vi "自动测试计算误差.vi"(8 "反馈值":dbl, 9 "输入值":dbl, 11 "DSP_OR_AD":i32) -> (1 "误差":dbl, 3 "合格？":bool)   [LabVIEW 2010]
uses:
  全局量/全局_配置.vi
panel:
  in  "AD量程":dbl
  in  "误差合格范围":dbl
  in  "DSP量程":dbl
  # "0为DSP，1为AD"
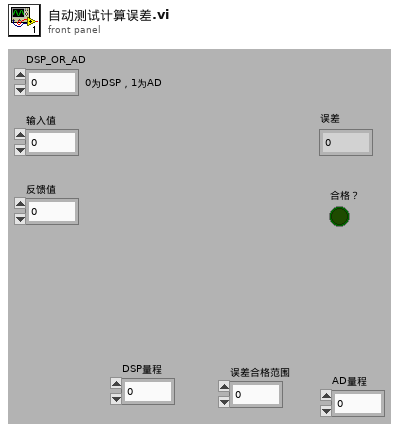
[diagram p1: front panel]
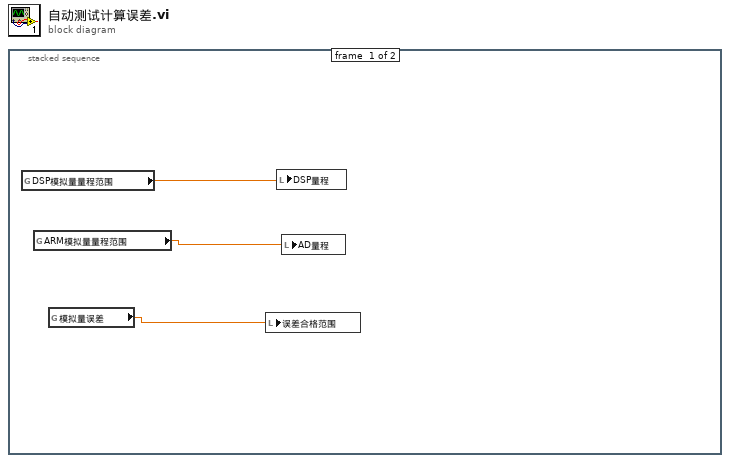
[diagram p0: block diagram]
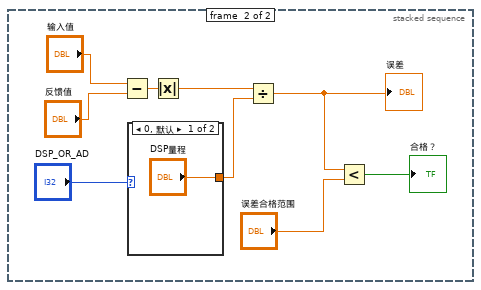
[diagram p2: hidden frame]
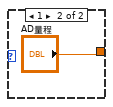
[diagram p3: hidden frame]
diagram:
  n1 = stacked-sequence {
    frame #0 {
      n2 = global read "全局_配置.vi" "DSP模拟量量程范围"() -> (w2:dbl)
      n3 = global read "全局_配置.vi" "ARM模拟量量程范围"() -> (w1:dbl)
      n4 = global read "全局_配置.vi" "模拟量误差"() -> (w3:dbl)
      n5 = local write "误差合格范围"(w3) -> ()
      n6 = local write "DSP量程"(w2) -> ()
      n7 = local write "AD量程"(w1) -> ()
    }
    frame #1 {
      n8 = Subtract(x="输入值", y="反馈值") -> (x-y=w10:dbl)
      n9 = case shown="0, 默认" "DSP_OR_AD" {
        tunnel: ["DSP量程" "AD量程"] -> w7
        frame 0, Default {
        }
        frame 1 {
        }
      }
      n10 = Absolute Value(x=w10) -> (abs(x)=w9:dbl)
      n11 = Divide(x=w9, y=w7) -> (x/y=w4:dbl)
      "误差" <- w4
      n12 = Less?(x=w4, y="误差合格范围") -> (x < y?=→"合格？":bool)
    }
  }
